vi "Add Tree Entry to Map.vi"(6 "Parent (None)":string[](array[string]), 7 "Name Prefix (none)":string, 9 "Columns":string[](array[string]), 10 "Name":string, 11 "Map in":map{string[], T1}(c390)) -> (3 "Map":map{string[], T1}(c390), 4 "Hierarchy":string[](array[string]))   [LabVIEW 2020, in "VectoTools.lvlib" / "TelemetryDebug.lvclass"]
uses:
  TelemetryDebug.lvclass
  Tree Entry.ctl
  TelemetryDebug.lvclass/TelemetryDebug.ctl
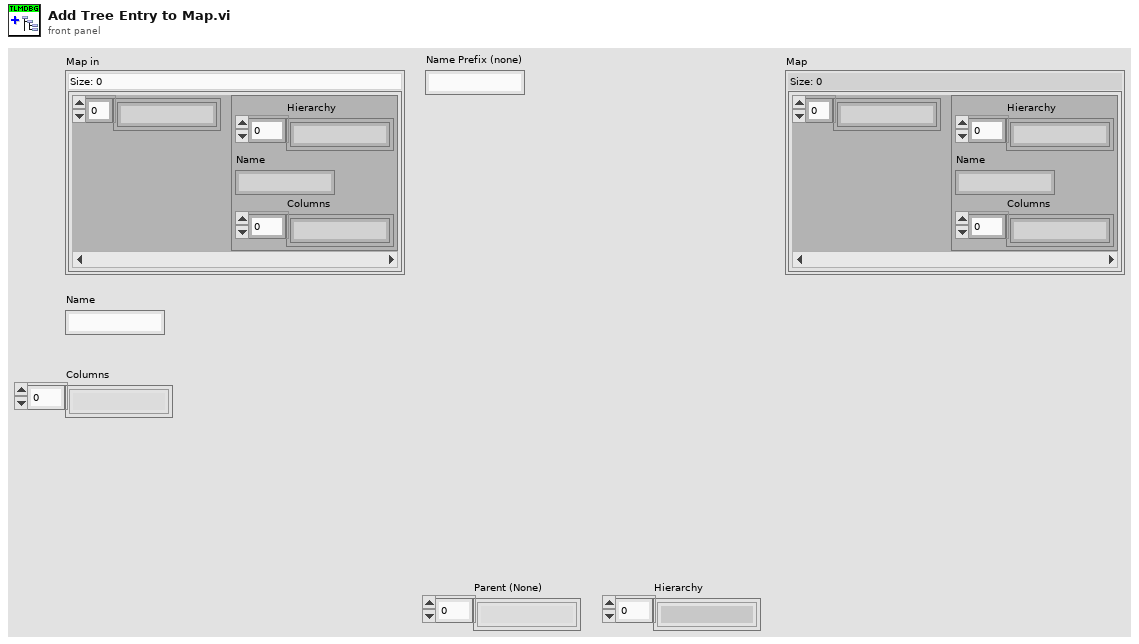
[diagram p1: front panel]
types:
  T1 = typedef "VectoTools.lvlib/TelemetryDebug.lvclass/Tree Entry.ctl" = cluster{"Hierarchy":string[], "Name":string, "Columns":string[]}
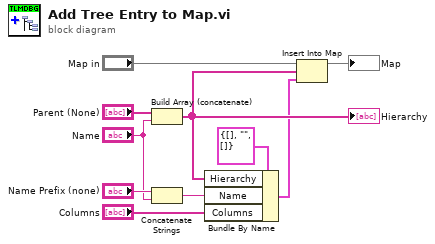
[diagram p0: block diagram]
diagram:
  n1 = Build Array (concatenate)("Parent (None)", "Name") -> (w6:string[])
  "Hierarchy" <- w6
  n2 = Concatenate Strings("Name Prefix (none)", "Name") -> (w1:string)
  n3 = Bundle By Name(cluster=T1 {"Hierarchy"=[], "Name"="", "Columns"=[]} ("Tree Entry"), "Hierarchy"=w6, "Name"=w1, "Columns"="Columns") -> (w5:T1)
  n4 = Insert Into Map(map in="Map in", key=w6, value=w5) -> (map out=→"Map":map{string[], T1})  [unwired: 2 out]
